vi "Generate Monitor Boundaries.vi"(6 "Starting Address Offset":u16 format="%04x", 8 "error in (no error)":errorcluster, 11 "Bus Monitor in":refnum<class "Bus Monitor.lvclass">) -> (0 "error out":errorcluster, 1 "Bus B Bounds":u16[](array[numeric])=[2048, 2048, 3447, 3446, 3448, 3448, 15697, 15696] format="%04x", 2 "Bus A Bounds":u16[](array[numeric])=[2048, 2048, 3447, 3446, 3448, 3448, 15697, 15696] format="%04x", 3 "Bus Monitor out":refnum<class "Bus Monitor.lvclass">)   [LabVIEW 2016, in "BCI-1553 API.lvlib" / "Bus Monitor.lvclass"]
doc: "Generates the Bus A and Bus B memory boundaries for storing records."
uses:
  Bus Monitor.lvclass
panel:
  out "Data 3":u16=1
  out "Data 2":u16=1
  out "Data 1":u16=1
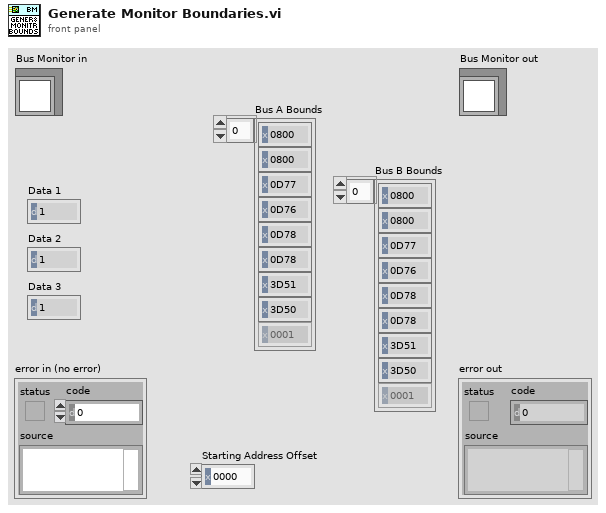
[diagram p1: front panel]
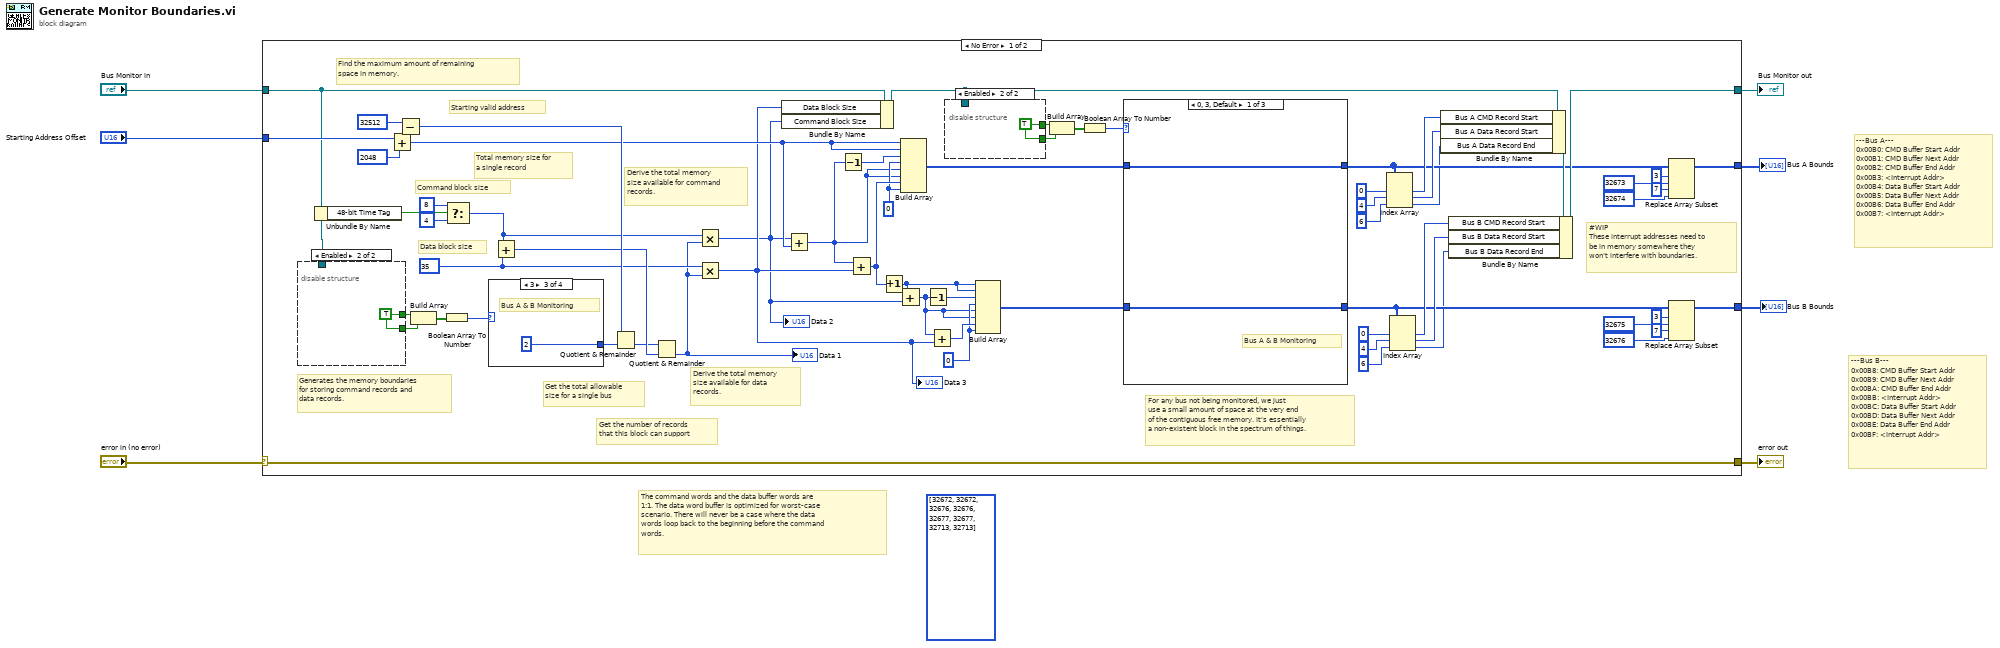
[diagram p0: block diagram]
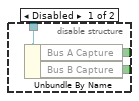
[diagram p2: hidden frame]
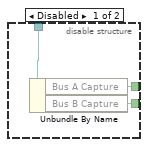
[diagram p3: hidden frame]
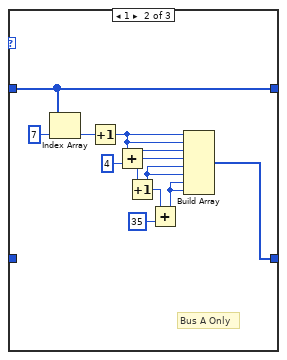
[diagram p4: hidden frame]
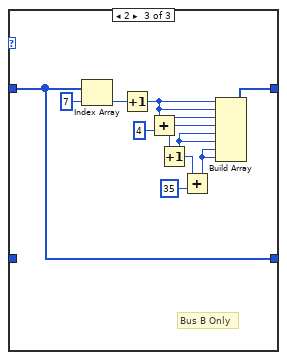
[diagram p5: hidden frame]
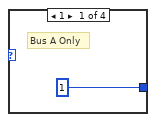
[diagram p6: hidden frame]
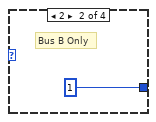
[diagram p7: hidden frame]
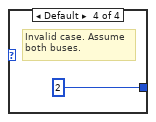
[diagram p8: hidden frame]
diagram:
  (unwired) u16[] [32672, 32672, 32676, 32676, 32677, 32677, 32713, 32713] ("Bus A Bounds")
  # "The command words and the data buffer words are\n1:1. The data word buffer is optimized for worst-case\nscenario. There will never be a case where the data\nwords loop back to the beginning before the command\nwords."
  # "---Bus B---\n0x00B8: CMD Buffer Start Addr\n0x00B9: CMD Buffer Next Addr\n0x00BA: CMD Buffer End Addr\n0x00BB: <Interrupt Addr>\n0x00BC: Data Buffer Start Addr\n0x00BD: Data Buffer Next Addr\n0x00BE: Data Buffer End Addr\n0x00BF: <Interrupt Addr>"
  # "---Bus A---\n0x00B0: CMD Buffer Start Addr\n0x00B1: CMD Buffer Next Addr\n0x00B2: CMD Buffer End Addr\n0x00B3: <Interrupt Addr>\n0x00B4: Data Buffer Start Addr\n0x00B5: Data Buffer Next Addr\n0x00B6: Data Buffer End Addr\n0x00B7: <Interrupt Addr>"
  n1 = case shown="No Error" "error in (no error)" {
    selector: "error in (no error)" -> [w71 w107]
    tunnel: [w71 w107] -> w6
    tunnel: [w44 w106] -> w5
    tunnel: "Bus Monitor in" -> [w39 w106]
    tunnel: "Starting Address Offset" -> [w69 _]
    tunnel: [w29 _] -> w3
    tunnel: [w27 _] -> w2
    frame No Error {
      w16 = u16 0 ("element")
      w17 = u16 0 ("element")
      w57 = u16 35 ("Numeric")
      # "#WIP\nThese interrupt addresses need to\nbe in memory somewhere they\nwon't interfere with boundaries."
      # "For any bus not being monitored, we just\nuse a small amount of space at the very end\nof the contiguous free memory. It's essentially\na non-existent block in the spectrum of things."
      # "Generates the memory boundaries\nfor storing command records and \ndata records."
      # "Starting valid address"
      # "Derive the total memory\nsize available for data\nrecords."
      # "Derive the total memory\nsize available for command\nrecords."
      # "Get the number of records\nthat this block can support"
      # "Get the total allowable\nsize for a single bus"
      # "Total memory size for\na single record"
      # "Data block size"
      # "Command block size"
      # "Find the maximum amount of remaining\nspace in memory."
      n2 = disable-structure shown="Enabled" {
        disable-tunnel: [w78 w79] -> w67
        disable-tunnel: [w77 w79] -> w66
        disable-tunnel: w39 -> [w76 _]
        frame Disabled {
          n3 = Unbundle By Name(w76) -> ("Bus A Capture"=w78:bool, "Bus B Capture"=w77:bool)
        }
        frame Enabled {
          w79 = TRUE ("Bus A Capture")
        }
      }
      n4 = Unbundle By Name(w39) -> ("48-bit Time Tag"=w53:bool)
      n5 = Add(x=w69, y=u16 2048 ("Numeric")) -> (x+y=w56:u16)
      n6 = Subtract(x=u16 32512 ("Numeric"), y=w56) -> (x-y=w63:u16)
      n7 = Build Array(w67, w66) -> (w65:bool[])
      n8 = Boolean Array To Number(Boolean array=w65) -> (number=w64:u32)
      n9 = Select(t=u16 8 ("Numeric"), s=w53, f=u16 4 ("Numeric")) -> (s? t:f=w58:u16)
      n10 = case shown="3" w64 {
        tunnel: [u16 1 u16 1 u16 2 u16 2] -> w62
        frame 1 {
          # "Bus A Only"
        }
        frame 2 {
          # "Bus B Only"
        }
        frame 3 {
          # "Bus A & B Monitoring"
        }
        frame Default {
          # "Invalid case. Assume\nboth buses."
        }
      }
      n11 = Add(x=w58, y=w57) -> (x+y=w59:u16)
      n12 = Quotient & Remainder(x=w63, y=w62) -> (floor(x/y)=w54:u16)  [unwired: 1 out]
      n13 = Quotient & Remainder(x=w54, y=w59) -> (floor(x/y)=w52:u16)  [unwired: 1 out]
      "Data 1" <- w52
      n14 = Multiply(x=w58, y=w52) -> (x*y=w36:u16)
      "Data 2" <- w36
      n15 = Multiply(x=w57, y=w52) -> (x*y=w37:u16)
      "Data 3" <- w37
      n16 = Bundle By Name(cluster=w39, "Data Block Size"=w37, "Command Block Size"=w36) -> (w38:refnum<class "Bus Monitor.lvclass">)
      n17 = Add(x=w36, y=w56) -> (x+y=w14:u16)
      n18 = Decrement(x=w14) -> (x-1=w15:u16)
      n19 = Add(x=w14, y=w37) -> (x+y=w35:u16)
      n20 = Increment(x=w35) -> (x+1=w55:u16)
      n21 = Add(x=w55, y=w36) -> (x+y=w12:u16)
      n22 = Build Array(w56, w56, w15, w17, w14, w14, w35, w17) -> (w48:u16[])
      n23 = Decrement(x=w12) -> (x-1=w13:u16)
      n24 = Add(x=w12, y=w37) -> (x+y=w34:u16)
      n25 = disable-structure shown="Enabled" {
        disable-tunnel: [w74 w75] -> w50
        disable-tunnel: [w73 w75] -> w49
        disable-tunnel: w38 -> [w72 _]
        frame Disabled {
          n26 = Unbundle By Name(w72) -> ("Bus A Capture"=w74:bool, "Bus B Capture"=w73:bool)
        }
        frame Enabled {
          w75 = TRUE ("Bus A Capture")
        }
      }
      n27 = Build Array(w55, w55, w13, w16, w12, w12, w34, w16) -> (w47:u16[])
      n28 = Build Array(w50, w49) -> (w51:bool[])
      n29 = Boolean Array To Number(Boolean array=w51) -> (number=w46:u32)
      n30 = case shown="0, 3, Default" w46 {
        tunnel: w48 -> [w81 w91 w94]
        tunnel: w47 -> [w80 _ _]
        tunnel: [w81 w91 w93] -> w28
        tunnel: [w80 w83 w94] -> w26
        frame 0, 3, Default {
          # "Bus A & B Monitoring"
        }
        frame 1 {
          # "Bus A Only"
          n31 = Index Array(array=w91, index=7) -> (element=w90:u16)
          n32 = Increment(x=w90) -> (x+1=w89:u16)
          n33 = Add(x=w89, y=u16 4) -> (x+y=w86:u16)
          n34 = Increment(x=w86) -> (x+1=w85:u16)
          n35 = Add(x=w85, y=u16 35) -> (x+y=w84:u16)
          n36 = Build Array(w89, w89, w86, w86, w85, w85, w84, w84) -> (w83:u16[])
        }
        frame 2 {
          # "Bus B Only"
          n37 = Index Array(array=w94, index=7) -> (element=w101:u16)
          n38 = Increment(x=w101) -> (x+1=w100:u16)
          n39 = Add(x=w100, y=u16 4) -> (x+y=w97:u16)
          n40 = Increment(x=w97) -> (x+1=w96:u16)
          n41 = Add(x=w96, y=u16 35) -> (x+y=w95:u16)
          n42 = Build Array(w100, w100, w97, w97, w96, w96, w95, w95) -> (w93:u16[])
        }
      }
      n43 = Index Array(array=w28, index #1=0 ("index"), index #2=4 ("index"), index #3=6 ("index")) -> (element #1=w33:u16, element #2=w32:u16, element #3=w10:u16)
      n44 = Index Array(array=w26, index #1=0 ("index"), index #2=4 ("index"), index #3=6 ("index")) -> (element #1=w31:u16, element #2=w30:u16, element #3=w8:u16)
      n45 = Bundle By Name(cluster=w38, "Bus A CMD Record Start"=w33, "Bus A Data Record Start"=w32, "Bus A Data Record End"=w10) -> (w45:refnum<class "Bus Monitor.lvclass">)
      n46 = Bundle By Name(cluster=w45, "Bus B CMD Record Start"=w31, "Bus B Data Record Start"=w30, "Bus B Data Record End"=w8) -> (w44:refnum<class "Bus Monitor.lvclass">)
      n47 = Replace Array Subset(array=w28, new element #1=u16 32673 ("Numeric"), index #1=3 ("index"), new element #2=u16 32674 ("Numeric"), index #2=7 ("index")) -> (w29:u16[])
      n48 = Replace Array Subset(array=w26, new element #1=u16 32675 ("Numeric"), index #1=3 ("index"), new element #2=u16 32676 ("Numeric"), index #2=7 ("index")) -> (w27:u16[])
    }
    frame Error {
    }
  }
  "error out" <- w6
  "Bus Monitor out" <- w5
  "Bus B Bounds" <- w2
  "Bus A Bounds" <- w3
